vi "Prefilter.Low Pass.vi"(8 "error in (no error)":errorcluster, 11 "Instrument.DAQ":refnum<class "Instrument.DAQ.lvclass">) -> (0 "error out":errorcluster, 3 "Instrument.DAQ out":refnum<class "Instrument.DAQ.lvclass">)   [LabVIEW 2019, in "Instrument.DAQ.lvclass"]
uses:
  Instrument.DAQ.lvclass
  Instrument.DAQ.lvclass/Instrument.DAQ.ctl
  <vilib>/addons/Digital Filter Design/Process.llb/DFD Filtering (Wfm NChan).vi
  <vilib>/addons/Digital Filter Design/NI_DigFilterLicensed.lvlib
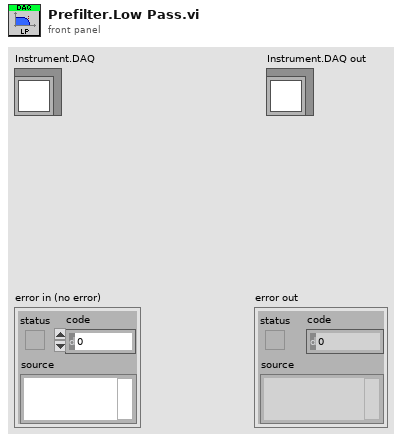
[diagram p1: front panel]
types:
  T1 = enum16{"Lowpass", "Highpass", "Bandpass", "Bandstop"}
  T2 = typedef "NI_DigFilterLicensed.lvlib/DFD Filter Obj.ctl" = cluster{"mSRate_Fs":dbl, "mSRate_Version":string, "mSRate_Comments":string, "mSRate_OrgCoef":T3, "mSRate_CurCoef":T3, "mSRate_Quantized?":bool, "mSRate_QCoef":T3, "mSRate_QSettings":T5[], "mSRate_Order":i32, "mSRate_Scaling":cluster{"mSRate_ScaleByPowerOf2?":bool, "mSRate_ScaleType":T7}}
  T3 = typedef "NI_DigFilterLicensed.lvlib/DFD Filter Coef.ctl" = cluster{"type":T4, "gain":dbl, "coef a (k)":dbl[], "coef b (v)":dbl[]}
  T4 = typedef "NI_DigFilterLicensed.lvlib/DFD Filter Structure Type Selector.ctl" = enum16{"Undefined", "FIR Direct Form", "FIR Direct Form Transposed", "FIR Symmetric", "FIR Antisymmetric", "IIR Direct Form I", "IIR Direct Form I Transposed", "IIR Direct Form II", "IIR Direct Form II Transposed", "IIR Cascaded Second Order Sections Form I", "IIR Cascaded Second Order Sections Form I Transposed", "IIR Cascaded Second Order Sections Form II", "IIR Cascaded Second Order Sections Form II Transposed", "Lattice Allpass (basic sections)", "Lattice Allpass (one multiplier sections)", "Lattice Allpass (normalized sections)", "Lattice AR (basic sections)", "Lattice AR (one multiplier sections)", "Lattice AR (normalized sections)", "Lattice MA (minimum phase)", "Lattice MA (maximum phase)", "Lattice ARMA (basic sections)", "Lattice ARMA (one multiplier sections)", "Lattice ARMA (normalized sections)"}
  T5 = typedef "NI_DigFilterLicensed.lvlib/dfd_Internal Quantization Settings.ctl" = cluster{"source":T6, "wl":i16, "iwl":i16, "overflow mode":enum16{"Saturation", "Wrap"}, "rounding mode":enum16{"Nearest", "Truncation"}, "signed?":bool}
  T6 = typedef "NI_DigFilterLicensed.lvlib/dfd_Internal Quantization Srcs.ctl" = u16
  T7 = typedef "NI_DigFilterLicensed.lvlib/DFD Coef Norm Type.ctl" = enum16{"No Norm", "Time Domain 1-Norm", "Time Domain 2-Norm", "Time Domain Inf-Norm"}
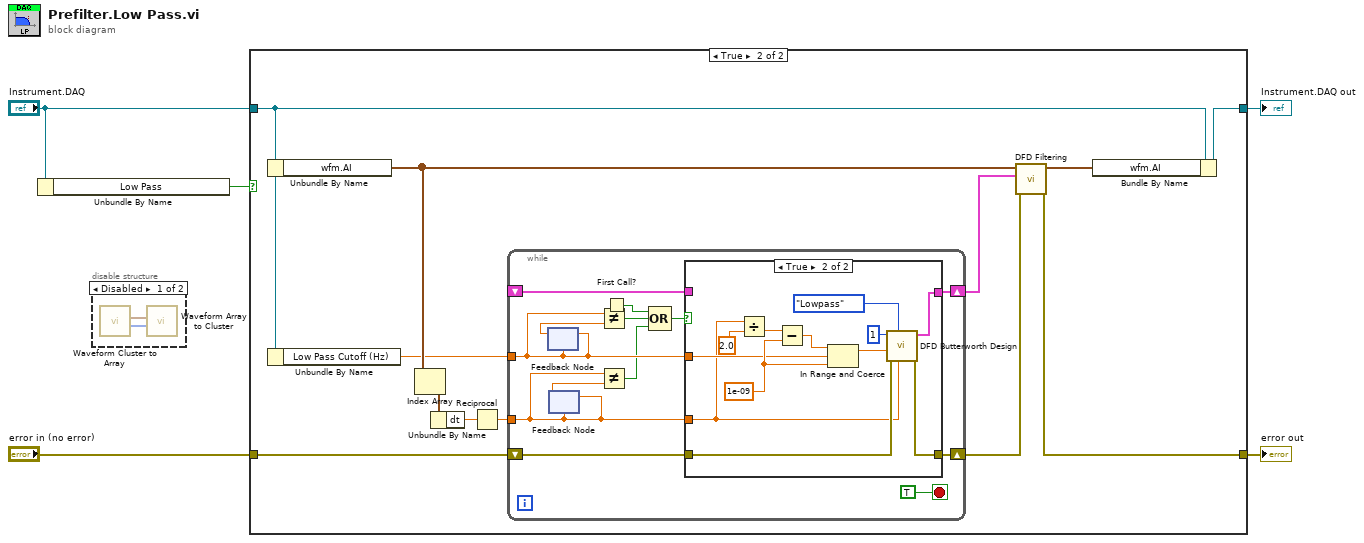
[diagram p0: block diagram]
diagram:
  n1 = Unbundle By Name("Instrument.DAQ") -> ("Low Pass"=w1:bool)
  n2 = disable-structure shown="Disabled" {
    frame Disabled {
      n3 = call "Waveform Cluster to Array.vi"() -> ("Lengths"=w6:i32[], "Concatenated Waveforms"=w7:waveform(dbl)[])  [unwired: 10 in]
      n4 = call "Waveform Array to Cluster.vi"("Lengths"=w6, "Concatenated Waveforms"=w7) -> ()  [unwired: 9 in, 1 out]
    }
    frame Enabled {
    }
  }
  n5 = case shown="True" w1 {
    tunnel: "error in (no error)" -> [w8 w18]
    tunnel: [w8 w11] -> w4
    tunnel: "Instrument.DAQ" -> [w9 w14]
    tunnel: [w9 w16] -> w3
    frame False {
    }
    frame True {
      n6 = Unbundle By Name(w14) -> ("wfm.AI"=w17:waveform(dbl)[])
      n7 = Unbundle By Name(w14) -> ("Low Pass Cutoff (Hz)"=w13:dbl)
      n8 = Index Array(array=w17) -> (element=w20:waveform(dbl))  [unwired: 1 in]
      n9 = Unbundle By Name(w20) -> ("dt"=w21:dbl)
      n10 = Reciprocal(x=w21) -> (1/x=w12:dbl)
      n11 = while {
        tunnel: w13 -> [w30]
        tunnel: w12 -> [w28]
        shift-right: [w32] -> w10
        shift-left: w18 -> [w33]
        shift-right: [w34] -> w19
        shift-left: _ -> [w24]
        stop <- TRUE stop-if-true
        n12 = feedback-in #1(w30) -> ()
        n13 = feedback #1(w30) -> (w22:dbl)
        n14 = feedback #2(w28) -> (w29:dbl)
        n15 = feedback-in #2(w28) -> ()
        n16 = Not Equal?(x=w30, y=w22) -> (x != y?=w26:bool)
        n17 = Not Equal?(x=w28, y=w29) -> (x != y?=w25:bool)
        n18 = First Call?() -> (First Call?: T/F=w27:bool)
        n19 = Compound Arithmetic op=OR(w27, w26, w25) -> (w23:bool)
        n20 = case shown="True" w23 {
          tunnel: [w36 w37] -> w34
          tunnel: w33 -> [w35 w47]
          tunnel: [w35 w40] -> w32
          tunnel: w30 -> [_ w39]
          tunnel: w28 -> [_ w38]
          tunnel: w24 -> [w36 _]
          frame False {
          }
          frame True {
            w42 = 1e-09 ("lower limit")
            n21 = Divide(x=w38, y=2.0 ("lower limit")) -> (x/y=w43:dbl)
            n22 = Subtract(x=w43, y=w42) -> (x-y=w41:dbl)
            n23 = In Range and Coerce(upper limit=w41, x=w39, lower limit=w42) -> (coerced(x)=w44:dbl)  [unwired: 1 out]
            n24 = call <vilib>:"DFD Butterworth Design.vi"("fs [Hz]"=w38, "filter type"=T1."Lowpass", "error in (no error)"=w47, "low cutoff freq [Hz]"=w44, "order"=1) -> ("error out"=w40:errorcluster, "filter out"=w37:T2)  [unwired: 5 in]
          }
        }
      }
      n25 = call-poly <vilib>:"DFD Filtering.vi"("error in (no error)"=w10, "filter"=w19, "signal in"=w17) -> ("error out"=w11:errorcluster, "signal out"=w15:waveform(dbl)[])  [unwired: 7 in]
      n26 = Bundle By Name(cluster=w14, "wfm.AI"=w15) -> (w16:refnum<class "Instrument.DAQ.lvclass">)
    }
  }
  "error out" <- w4
  "Instrument.DAQ out" <- w3
